vi "FPGA_M_test.vi"() -> ()   [LabVIEW 2018]
uses:
  Model/States.ctl
panel:
  out "Waveform Chart":u32(graph)
  out "dt":u32
  out "busy":bool
  in  "stop":bool
  in  "setpoint":i16
  out "fpga rt loop":i32
  out "States":T1 format="%.4f"
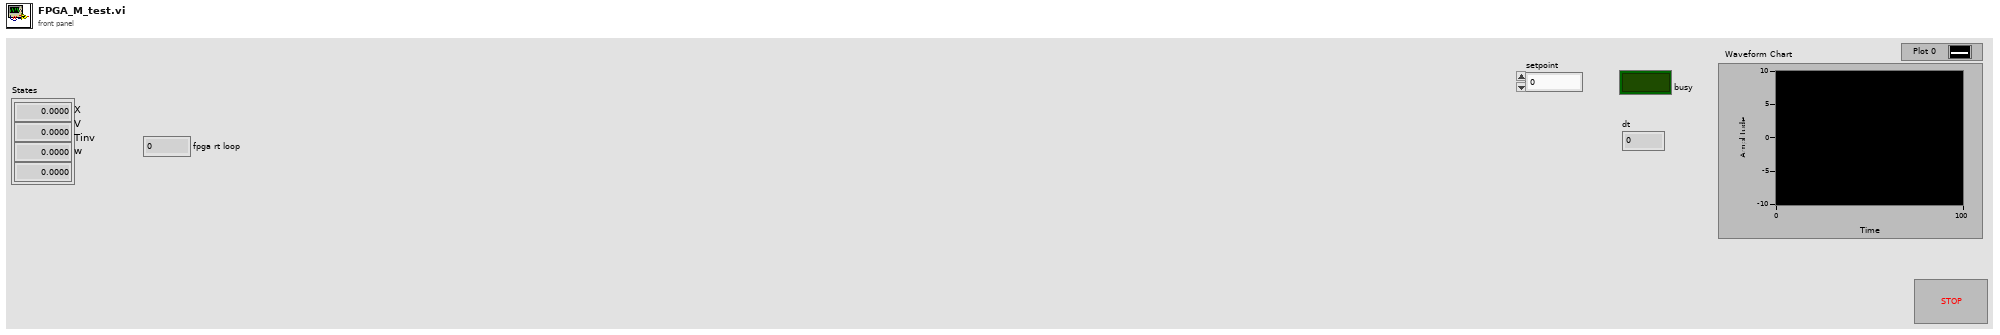
[diagram p1: front panel]
types:
  T1 = typedef "States.ctl" = dbl[]
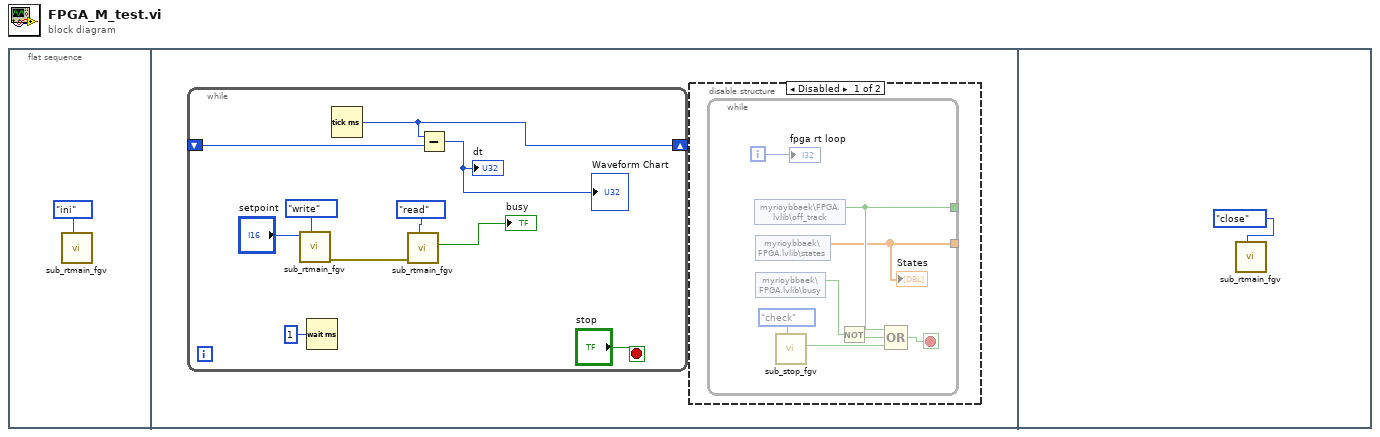
[diagram p0: block diagram]
diagram:
  n1 = flat-sequence {
    frame #0 {
      n2 = call "sub_rtmain_fgv.vi"("cmd"=enum16{"ini", "read", "write", "close"}."ini") -> ()  [unwired: 7 in, 4 out]
    }
    frame #1 {
      n3 = while {
        shift-right: [w4] -> _
        shift-left: _ -> [w3]
        stop <- "stop" stop-if-true
        n4 = call "sub_rtmain_fgv.vi"("cmd"=enum16{"ini", "read", "write", "close"}."write", "setpoint"="setpoint") -> ("error out"=w6:errorcluster)  [unwired: 6 in, 3 out]
        n5 = Wait (ms)(milliseconds to wait=u32 1) -> ()  [unwired: 1 out]
        n6 = Tick Count (ms)() -> (millisecond timer value=w4:u32)
        n7 = call "sub_rtmain_fgv.vi"("cmd"=enum16{"ini", "read", "write", "close"}."read", "error in"=w6) -> ("busy"=→"busy":bool)  [unwired: 6 in, 3 out]
        n8 = Subtract(x=w4, y=w3) -> (x-y=→"dt" →"Waveform Chart":u32)
      }
      n9 = disable-structure shown="Disabled" {
        frame Disabled {
          n10 = while {
            tunnel: [w15] -> _
            tunnel: [w12] -> _
            i -> [w19]
            stop <- w16 stop-if-true
            n11 = shared-variable "myrioybbaek\\FPGA.lvlib\\off_track"() -> (w15:bool)  [unwired: 1 in, 1 out]
            n12 = shared-variable "myrioybbaek\\FPGA.lvlib\\states"() -> (w12:dbl[])  [unwired: 1 in, 1 out]
            "States" <- w12
            n13 = shared-variable "myrioybbaek\\FPGA.lvlib\\busy"() -> (w14:bool)  [unwired: 1 in, 1 out]
            n14 = call "sub_stop_fgv.vi"("cmd"=enum16{"ini", "check", "stop"}."check") -> ("status"=w17:bool)  [unwired: 10 in]
            n15 = Not(x=w14) -> (.not. x?=w13:bool)
            n16 = Compound Arithmetic op=OR(w15, w13, w17) -> (w16:bool)
            "fpga rt loop" <- w19
          }
        }
        frame Enabled {
        }
      }
    }
    frame #2 {
      n17 = call "sub_rtmain_fgv.vi"("cmd"=enum16{"ini", "read", "write", "close"}."close") -> ()  [unwired: 7 in, 4 out]
    }
  }
